vi "Poll Cancelled.vi"(8 "error in (no error)":errorcluster, 11 "Promise in":refnum<class "Promise.lvclass">) -> (0 "error out":errorcluster, 2 "Cancelled":bool, 3 "Promise out":refnum<class "Promise.lvclass">)   [LabVIEW 2017, in "Futures.lvlib" / "Promise.lvclass"]
doc: "Poll for the cancelled flag. If this returns true - it means that there is no need to continue the task or resolve the promise."
uses:
  Promise.lvclass
  Promise.lvclass/Promise.ctl
  Task/Task.lvclass
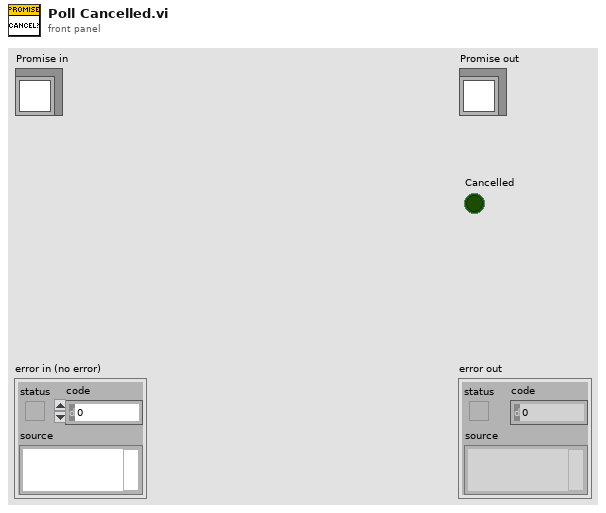
[diagram p1: front panel]
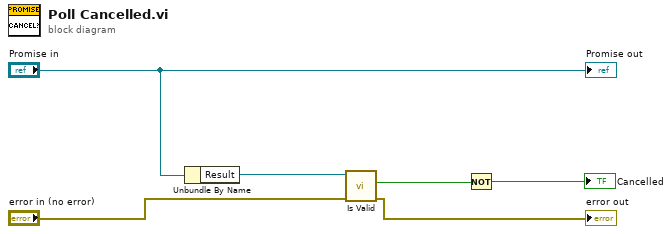
[diagram p0: block diagram]
diagram:
  n1 = Unbundle By Name("Promise in") -> ("Result"=w1:refnum<class "Task.lvclass">)
  n2 = call "Is Valid.vi"("error in (no error)"="error in (no error)", "Result in"=w1) -> ("error out"=→"error out":errorcluster, "Valid"=w2:bool)  [unwired: 7 in, 1 out]
  n3 = Not(x=w2) -> (.not. x?=→"Cancelled":bool)
  "Promise out" <- "Promise in"
